vi "GenerateMultiple3DPlot.vi"(8 "error in":errorcluster, 10 "3D Array":cluster{"X":dbl[], "Y":dbl[], "Z":dbl[]}[](array[cluster]), 11 "3D Scatter":refnum<class "3D Plot Datatype.lvclass">[](array[class])) -> (0 "error out":errorcluster, 3 "3D Scatter Out":refnum<class "3D Plot Datatype.lvclass">[](array[class]))   [LabVIEW 2020]
doc: "Generate multiple plots for the same graph"
uses:
  <vilib>/Math Plots/3D Math Plots/3D Plot/3D Plot Datatype/3D Plot Datatype.lvclass
  <vilib>/Math Plots/3D Math Plots/3D Scatter/3D Scatter Datatype/Public/Plot Helper (Vector).vi
  <vilib>/Math Plots/3D Math Plots/3D Scatter/3D Scatter Datatype/3D Scatter Datatype.lvclass
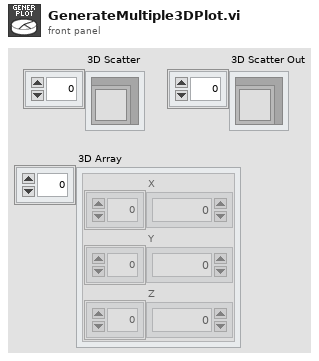
[diagram p1: front panel]
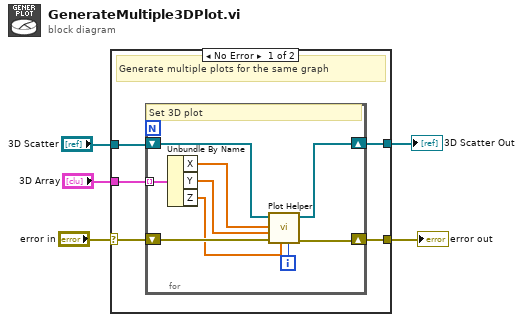
[diagram p0: block diagram]
diagram:
  n1 = case shown="No Error" "error in" {
    selector: "error in" -> [w10 w21]
    tunnel: [w8 w21] -> w3
    tunnel: [w9 w20] -> w5
    tunnel: "3D Scatter" -> [w7 w20]
    tunnel: "3D Array" -> [w6 _]
    frame No Error {
      # "Generate multiple plots for the same graph"
      n2 = for {
        tunnel: w6 -> [w17] mode=indexing
        shift-right: [w11] -> w9
        shift-left: w7 -> [w12]
        shift-right: [w18] -> w8
        shift-left: w10 -> [w19]
        i -> [w13]
        # "Set 3D plot"
        n3 = Unbundle By Name(w17) -> ("X"=w16:dbl[], "Y"=w15:dbl[], "Z"=w14:dbl[])
        n4 = call-poly <vilib>:"Plot Helper.vi"("Plot ID"=w13, "z vector"=w14, "error in (no error)"=w19, "y vector"=w15, "x vector"=w16, "3D Plot lvclass Array in"=w12) -> ("error out"=w18:errorcluster, "3D Plot lvclass Array out"=w11:refnum<class "3D Plot Datatype.lvclass">[])  [unwired: 4 out]
      }
    }
    frame Error {
    }
  }
  "3D Scatter Out" <- w5
  "error out" <- w3
